vi "_Ramp Generator.vi"() -> ()   [LabVIEW 2013]
panel:
  in  "Stop Button":bool
  out "VISA Refnum out":refnum<visa-resource-name>
  out "concatenated string":string
  out "error out":errorcluster
  in  "VISA resource name":refnum<visa-resource-name>
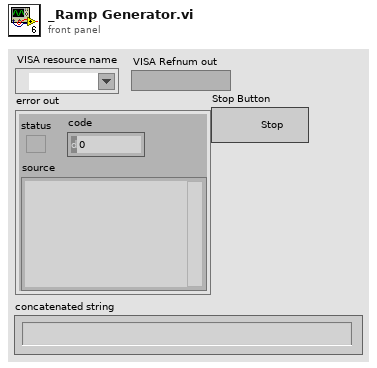
[diagram p1: front panel]
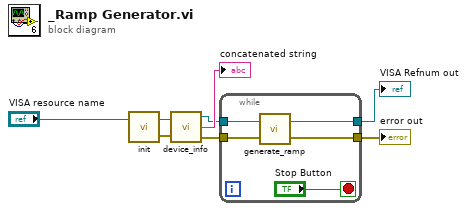
[diagram p0: block diagram]
diagram:
  n1 = call "init.vi"("VISA Refnum in"="VISA resource name") -> ("error out"=w6:errorcluster, "VISA Refnum out"=w7:refnum<visa-resource-name>)  [unwired: 1 in]
  n2 = call "device_info.vi"("VISA Refnum in"=w7, "error in (no error)"=w6) -> ("VISA Refnum out"=w4:refnum<visa-resource-name>, "concatenated string"=→"concatenated string":string, "error out"=w3:errorcluster)
  n3 = while {
    tunnel: w4 -> [w13]
    tunnel: w3 -> [w12]
    tunnel: [w11] -> w2
    tunnel: [w10] -> w1
    stop <- "Stop Button" stop-if-true
    n4 = call "generate_ramp.vi"("error in (no error)"=w12, "VISA Refnum in"=w13) -> ("error out"=w10:errorcluster, "VISA Refnum out"=w11:refnum<visa-resource-name>)
  }
  "error out" <- w1
  "VISA Refnum out" <- w2
